vi "save_data (SubVI).vi"(0 "Scope True?":bool=TRUE, 1 "Refnum in":refnum<k20>, 2 "Sample rate scope":dbl format="%#_13g", 3 "Sample rate":dbl format="%#_13g", 4 "error in":errorcluster, 5 "Filename":path, 6 "environ cluster":cluster{dbl[], dbl[]}, 7 "data":i16[][](array[numeric]), 8 "Process list":T1) -> ()   [LabVIEW 2018]
uses:
  <vilib>/addons/h5labview2/file/H5Fmode.ctl
  <vilib>/Utility/error.llb/Error Cluster From Error Code.vi
  <vilib>/rvi/errors/niLvFpgaAdjustHostInterfaceError.vi
  <vilib>/addons/h5labview2/base/lib_path.vi
  <vilib>/addons/h5labview2/base/H5Equery.vi
  <vilib>/rvi/interface/nirviReadWriteControl/nirviReadWriteControl.xnode
  FPGA code/FPGA Bitfiles/Microspherefeedb_FPGATarget2_(FPGA)PIDXYZlase_Y-TtBVY85Jw.lvbitx
  <vilib>/addons/h5labview2/dataset/H5Dwrite.llb/H5Dwrite.xnode
  <vilib>/addons/h5labview2/attrib/H5Awrite.llb/H5Awrite.xnode
  <vilib>/addons/h5labview2/base/hid_t.ctl
  <vilib>/addons/h5labview2/file/H5F.lvlib
  <vilib>/addons/h5labview2/group/H5G.lvlib
  NiFpgaLv.dll
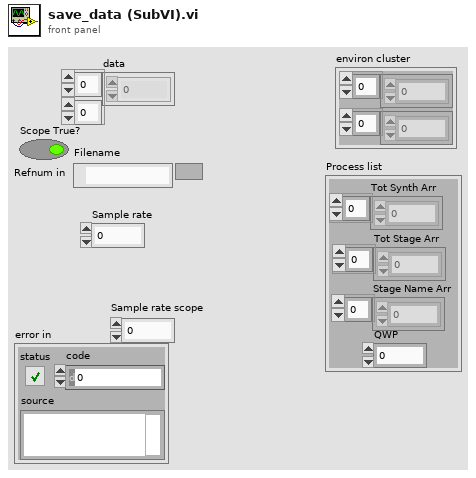
[diagram p1: front panel]
types:
  T1 = cluster{"Tot Synth Arr":dbl[], "Tot Stage Arr":dbl[], "Stage Name Arr":dbl[], "QWP":dbl}
  T2 = typedef "H5F.lvlib/H5Fmode.ctl" = enum16{"read-only", "read-write", "overwrite", "create new", "open or create"}
  T3 = typedef "hid_t.ctl" = i32
  T4 = cluster{"Sample rate":dbl, dbl, dbl[], dbl[], "QWP":dbl, "Tot Stage Arr":dbl[], sgl[]}
  T5 = cluster{"Sample rate":dbl, dbl, dbl[], dbl[], "QWP":dbl, "Tot Stage Arr":dbl[], "Sample rate scope":dbl}
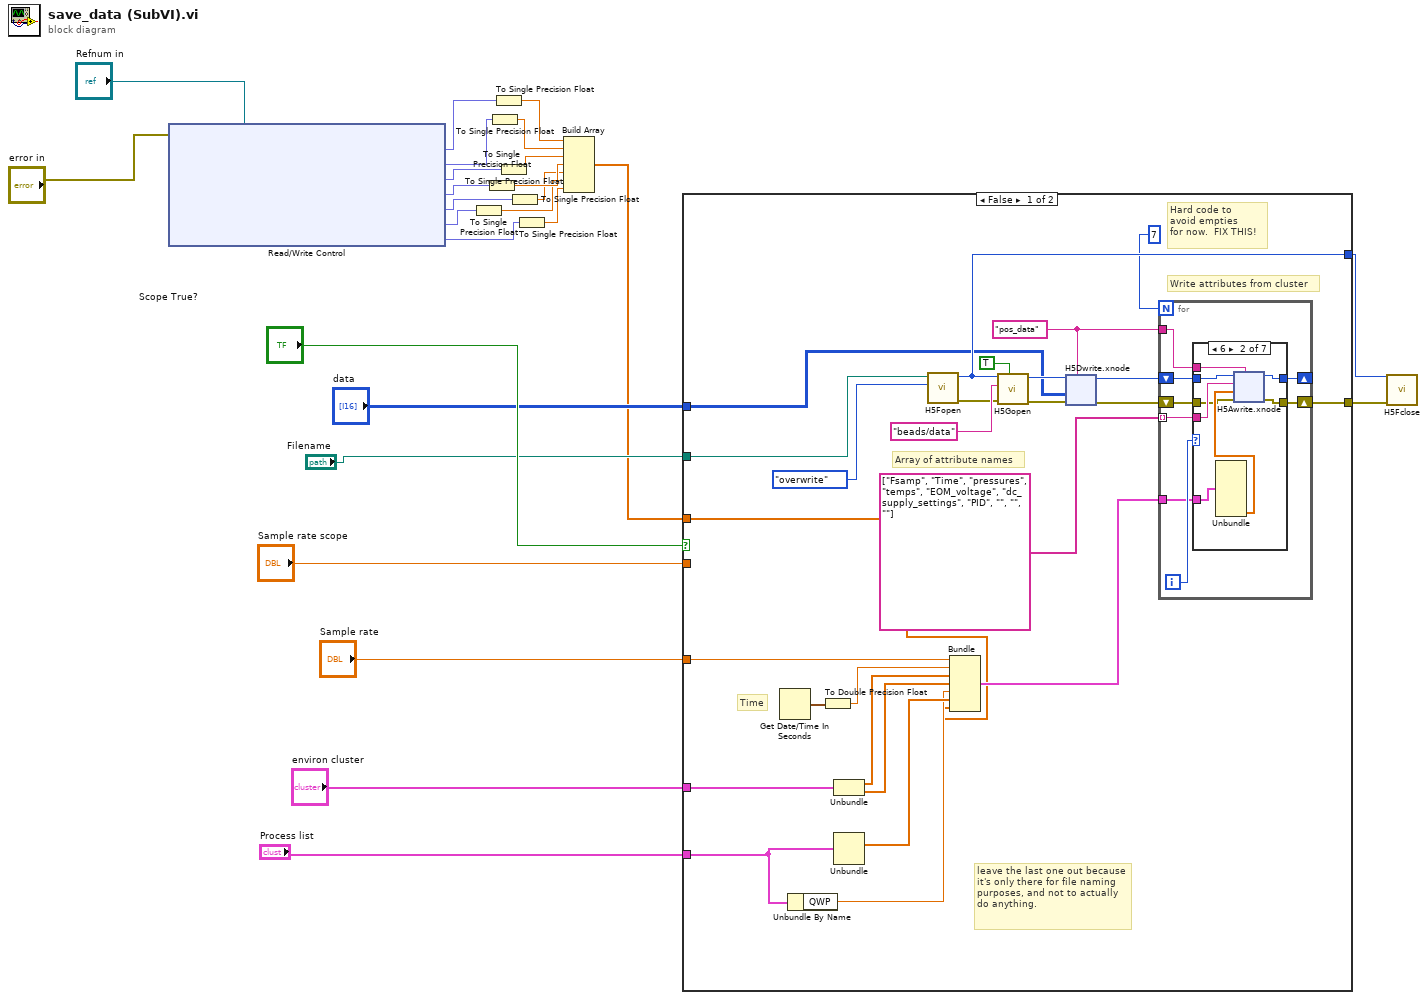
[diagram p0: block diagram]
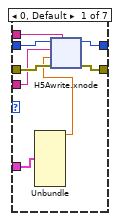
[diagram p2: hidden frame]
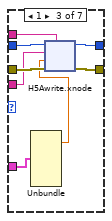
[diagram p3: hidden frame]
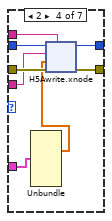
[diagram p4: hidden frame]
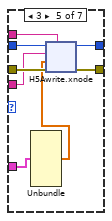
[diagram p5: hidden frame]
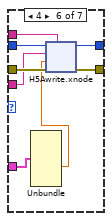
[diagram p6: hidden frame]
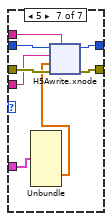
[diagram p7: hidden frame]
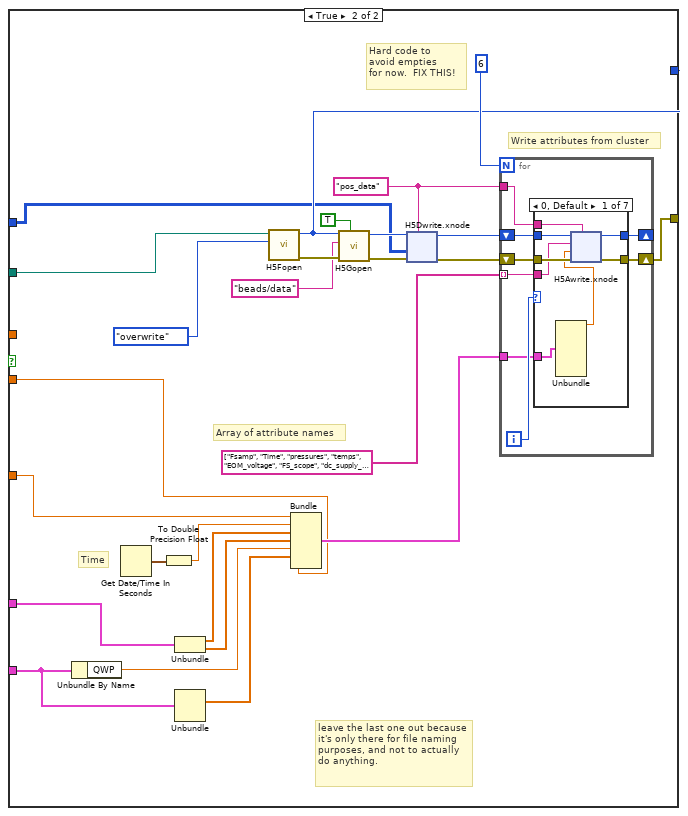
[diagram p8: hidden frame]
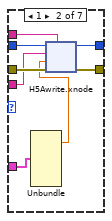
[diagram p9: hidden frame]
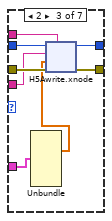
[diagram p10: hidden frame]
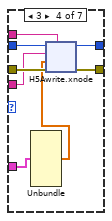
[diagram p11: hidden frame]
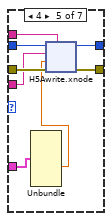
[diagram p12: hidden frame]
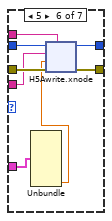
[diagram p13: hidden frame]
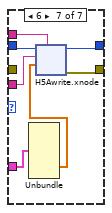
[diagram p14: hidden frame]
diagram:
  n1 = xnode "Read/Write Control"("FPGA VI Reference In"="Refnum in", "error in"="error in") -> ("dg X"=w14:fxp<+/-,24,12>, "ig X"=w12:fxp<+/-,24,-4>, "dg Y"=w10:fxp<+/-,24,12>, "ig Y"=w8:fxp<+/-,24,-4>, "pg Z"=w6:fxp<+/-,24,12>, "ig Z"=w4:fxp<+/-,24,-4>, "dg Z"=w2:fxp<+/-,24,12>)  [unwired: 2 out]
  n2 = To Single Precision Float(number=w4) -> (single precision float=w3:sgl)
  n3 = To Single Precision Float(number=w8) -> (single precision float=w7:sgl)
  n4 = To Single Precision Float(number=w12) -> (single precision float=w11:sgl)
  n5 = To Single Precision Float(number=w14) -> (single precision float=w13:sgl)
  n6 = To Single Precision Float(number=w10) -> (single precision float=w9:sgl)
  n7 = To Single Precision Float(number=w6) -> (single precision float=w5:sgl)
  n8 = To Single Precision Float(number=w2) -> (single precision float=w1:sgl)
  n9 = Build Array(w13, w11, w9, w7, w5, w3, w1) -> (w15:sgl[])
  n10 = case shown="False" "Scope True?" {
    tunnel: [w46 w275] -> w26
    tunnel: [w36 w276] -> w25
    tunnel: "Process list" -> [w32 w271]
    tunnel: "environ cluster" -> [w31 w272]
    tunnel: "Sample rate" -> [w30 w270]
    tunnel: "Filename" -> [w29 w273]
    tunnel: "data" -> [w28 w274]
    tunnel: "Sample rate scope" -> [_ w269]
    tunnel: w15 -> [w27 _]
    frame False {
      w52 = "pos_data" ("dataset name")
      # "leave the last one out because it's only there for file naming purposes, and not to actually do anything."
      # "Hard code to \navoid empties\nfor now.  FIX THIS!"
      # "Time"
      # "Array of attribute names"
      # "Write attributes from cluster"
      n11 = Get Date/Time In Seconds() -> (seconds since 1Jan1904=w48:timestamp)
      n12 = Unbundle By Name(w32) -> ("QWP"=w33:dbl)
      n13 = To Double Precision Float(number=w48) -> (double precision float=w41:dbl)
      n14 = Unbundle(w31) -> (w40:dbl[], w39:dbl[])
      n15 = Unbundle(w32) -> ("Tot Stage Arr"=w35:dbl[])  [unwired: 3 out]
      n16 = call <vilib>:"H5Fopen.vi"("mode (read-only)"=H5Fmode."overwrite", "path"=w29) -> ("error out"=w44:errorcluster, "ref out"=w36:T3)  [unwired: 8 in]
      n17 = Bundle("Sample rate"=w30, w41, w40, w39, "QWP"=w33, "Tot Stage Arr"=w35, w27) -> (w38:T4)  [unwired: 1 in]
      n18 = call <vilib>:"H5Gopen.vi"("create? (F)"=TRUE, "error in (no error)"=w44, "name"="beads/data", "ref in"=w36) -> ("error out"=w50:errorcluster, "group out"=w37:T3)  [unwired: 6 in]
      n19 = xnode "H5Dwrite.xnode"("dataset name"=w52, "error in (no error)"=w50, "data"=w28, "ref in"=w37) -> ("error out"=w49:errorcluster, "ref out"=w42:i32)  [unwired: 3 in, 1 out]
      n20 = for {
        N: 7 -> [_]
        tunnel: w52 -> [w60]
        shift-right: [w58] -> _
        shift-left: w42 -> [w55]
        shift-right: [w57] -> w46
        shift-left: w49 -> [w59]
        tunnel: string[] ["Fsamp", "Time", "pressures", "temps", "EOM_voltage", "dc_supply_settings", "PID", "", "", ""] -> [w56] mode=indexing
        tunnel: w38 -> [w53]
        i -> [w54]
        n21 = case shown="6" w54 {
          tunnel: w60 -> [w68 w95 w122 w149 w176 w203 w230]
          tunnel: w59 -> [w67 w89 w121 w148 w175 w202 w229]
          tunnel: [w66 w92 w120 w147 w174 w201 w228] -> w58
          tunnel: [w65 w88 w119 w146 w173 w200 w227] -> w57
          tunnel: w56 -> [w64 w94 w118 w145 w172 w199 w226]
          tunnel: w55 -> [w63 w93 w117 w144 w171 w198 w225]
          tunnel: w53 -> [w62 w91 w116 w143 w170 w197 w224]
          frame 0, Default {
            n22 = Unbundle(w62) -> ("Sample rate"=w61:dbl)  [unwired: 6 out]
            n23 = xnode "H5Awrite.xnode"("object name"=w68, "error in (no error)"=w67, "data"=w61, "attrib name"=w64, "ref in"=w63) -> ("error out"=w65:errorcluster, "ref out"=w66:T3)  [unwired: 2 in, 1 out]
          }
          frame 6 {
            n24 = Unbundle(w91) -> (w90:sgl[])  [unwired: 6 out]
            n25 = xnode "H5Awrite.xnode"("object name"=w95, "error in (no error)"=w89, "data"=w90, "attrib name"=w94, "ref in"=w93) -> ("error out"=w88:errorcluster, "ref out"=w92:T3)  [unwired: 2 in, 1 out]
          }
          frame 1 {
            n26 = Unbundle(w116) -> (w115:dbl)  [unwired: 6 out]
            n27 = xnode "H5Awrite.xnode"("object name"=w122, "error in (no error)"=w121, "data"=w115, "attrib name"=w118, "ref in"=w117) -> ("error out"=w119:errorcluster, "ref out"=w120:T3)  [unwired: 2 in, 1 out]
          }
          frame 2 {
            n28 = Unbundle(w143) -> (w142:dbl[])  [unwired: 6 out]
            n29 = xnode "H5Awrite.xnode"("object name"=w149, "error in (no error)"=w148, "data"=w142, "attrib name"=w145, "ref in"=w144) -> ("error out"=w146:errorcluster, "ref out"=w147:T3)  [unwired: 2 in, 1 out]
          }
          frame 3 {
            n30 = Unbundle(w170) -> (w169:dbl[])  [unwired: 6 out]
            n31 = xnode "H5Awrite.xnode"("object name"=w176, "error in (no error)"=w175, "data"=w169, "attrib name"=w172, "ref in"=w171) -> ("error out"=w173:errorcluster, "ref out"=w174:T3)  [unwired: 2 in, 1 out]
          }
          frame 4 {
            n32 = Unbundle(w197) -> ("QWP"=w196:dbl)  [unwired: 6 out]
            n33 = xnode "H5Awrite.xnode"("object name"=w203, "error in (no error)"=w202, "data"=w196, "attrib name"=w199, "ref in"=w198) -> ("error out"=w200:errorcluster, "ref out"=w201:T3)  [unwired: 2 in, 1 out]
          }
          frame 5 {
            n34 = Unbundle(w224) -> ("Tot Stage Arr"=w223:dbl[])  [unwired: 6 out]
            n35 = xnode "H5Awrite.xnode"("object name"=w230, "error in (no error)"=w229, "data"=w223, "attrib name"=w226, "ref in"=w225) -> ("error out"=w227:errorcluster, "ref out"=w228:T3)  [unwired: 2 in, 1 out]
          }
        }
      }
    }
    frame True {
      w277 = "pos_data" ("dataset name")
      # "leave the last one out because it's only there for file naming purposes, and not to actually do anything."
      # "Hard code to \navoid empties\nfor now.  FIX THIS!"
      # "Time"
      # "Array of attribute names"
      # "Write attributes from cluster"
      n36 = Unbundle By Name(w271) -> ("QWP"=w294:dbl)
      n37 = Get Date/Time In Seconds() -> (seconds since 1Jan1904=w281:timestamp)
      n38 = To Double Precision Float(number=w281) -> (double precision float=w287:dbl)
      n39 = Unbundle(w272) -> (w288:dbl[], w289:dbl[])
      n40 = Unbundle(w271) -> ("Tot Stage Arr"=w292:dbl[])  [unwired: 3 out]
      n41 = call <vilib>:"H5Fopen.vi"("mode (read-only)"=H5Fmode."overwrite", "path"=w273) -> ("error out"=w284:errorcluster, "ref out"=w276:T3)  [unwired: 8 in]
      n42 = Bundle("Sample rate"=w270, w287, w288, w289, "QWP"=w294, "Tot Stage Arr"=w292, "Sample rate scope"=w269) -> (w290:T5)  [unwired: 1 in]
      n43 = call <vilib>:"H5Gopen.vi"("create? (F)"=TRUE, "error in (no error)"=w284, "name"="beads/data", "ref in"=w276) -> ("error out"=w279:errorcluster, "group out"=w291:T3)  [unwired: 6 in]
      n44 = xnode "H5Dwrite.xnode"("dataset name"=w277, "error in (no error)"=w279, "data"=w274, "ref in"=w291) -> ("error out"=w280:errorcluster, "ref out"=w286:i32)  [unwired: 3 in, 1 out]
      n45 = for {
        N: 6 -> [_]
        tunnel: w277 -> [w302]
        shift-right: [w300] -> _
        shift-left: w286 -> [w297]
        shift-right: [w299] -> w275
        shift-left: w280 -> [w301]
        tunnel: string[] ["Fsamp", "Time", "pressures", "temps", "EOM_voltage", "FS_scope", "dc_supply_settings", "electrode_dc_vals", "stage_settings"] -> [w298] mode=indexing
        tunnel: w290 -> [w295]
        i -> [w296]
        n46 = case shown="0, Default" w296 {
          tunnel: w302 -> [w310 w337 w364 w391 w418 w445 w471]
          tunnel: w301 -> [w309 w336 w363 w390 w417 w444 _]
          tunnel: [w308 w335 w362 w389 w416 w443 w468] -> w300
          tunnel: [w307 w334 w361 w388 w415 w442 w467] -> w299
          tunnel: w298 -> [w306 w333 w360 w387 w414 w441 w470]
          tunnel: w297 -> [w305 w332 w359 w386 w413 w440 w469]
          tunnel: w295 -> [w304 w331 w358 w385 w412 w439 w466]
          frame 0, Default {
            n47 = Unbundle(w304) -> ("Sample rate"=w303:dbl)  [unwired: 6 out]
            n48 = xnode "H5Awrite.xnode"("object name"=w310, "error in (no error)"=w309, "data"=w303, "attrib name"=w306, "ref in"=w305) -> ("error out"=w307:errorcluster, "ref out"=w308:T3)  [unwired: 2 in, 1 out]
          }
          frame 1 {
            n49 = Unbundle(w331) -> (w330:dbl)  [unwired: 6 out]
            n50 = xnode "H5Awrite.xnode"("object name"=w337, "error in (no error)"=w336, "data"=w330, "attrib name"=w333, "ref in"=w332) -> ("error out"=w334:errorcluster, "ref out"=w335:T3)  [unwired: 2 in, 1 out]
          }
          frame 2 {
            n51 = Unbundle(w358) -> (w357:dbl[])  [unwired: 6 out]
            n52 = xnode "H5Awrite.xnode"("object name"=w364, "error in (no error)"=w363, "data"=w357, "attrib name"=w360, "ref in"=w359) -> ("error out"=w361:errorcluster, "ref out"=w362:T3)  [unwired: 2 in, 1 out]
          }
          frame 3 {
            n53 = Unbundle(w385) -> (w384:dbl[])  [unwired: 6 out]
            n54 = xnode "H5Awrite.xnode"("object name"=w391, "error in (no error)"=w390, "data"=w384, "attrib name"=w387, "ref in"=w386) -> ("error out"=w388:errorcluster, "ref out"=w389:T3)  [unwired: 2 in, 1 out]
          }
          frame 4 {
            n55 = Unbundle(w412) -> ("QWP"=w411:dbl)  [unwired: 6 out]
            n56 = xnode "H5Awrite.xnode"("object name"=w418, "error in (no error)"=w417, "data"=w411, "attrib name"=w414, "ref in"=w413) -> ("error out"=w415:errorcluster, "ref out"=w416:T3)  [unwired: 2 in, 1 out]
          }
          frame 5 {
            n57 = Unbundle(w439) -> ("Sample rate scope"=w438:dbl)  [unwired: 6 out]
            n58 = xnode "H5Awrite.xnode"("object name"=w445, "error in (no error)"=w444, "data"=w438, "attrib name"=w441, "ref in"=w440) -> ("error out"=w442:errorcluster, "ref out"=w443:T3)  [unwired: 2 in, 1 out]
          }
          frame 6 {
            n59 = Unbundle(w466) -> ("Tot Stage Arr"=w465:dbl[])  [unwired: 6 out]
            n60 = xnode "H5Awrite.xnode"("object name"=w471, "data"=w465, "attrib name"=w470, "ref in"=w469) -> ("error out"=w467:errorcluster, "ref out"=w468:T3)  [unwired: 3 in, 1 out]
          }
        }
      }
    }
  }
  n61 = call <vilib>:"H5Fclose.vi"("error in (no error)"=w26, "ref"=w25) -> ()  [unwired: 9 in, 1 out]
